vi "Get Typedef Path Dialog.vi"() -> (2 "Continue":bool, 3 "Stub VI Path":path, 5 "Typedef Path":path)   [LabVIEW 2012, in "Build Cluster of References__RCF.lvlib"]
uses:
  Build Cluster of References__RCF.lvlib
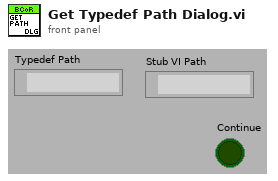
[diagram p1: front panel]
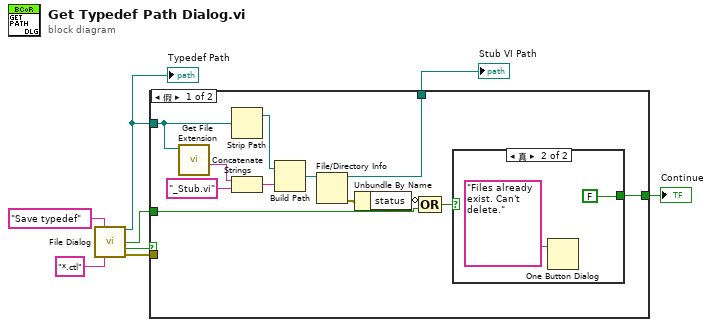
[diagram p0: block diagram]
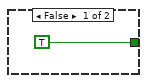
[diagram p2: hidden frame]
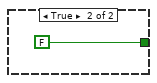
[diagram p3: hidden frame]
diagram:
  n1 = call "File Dialog"("prompt"="Save typedef", "pattern (all files)"="*.ctl") -> ("selected path"=w3:path, "exists"=w4:bool, "cancelled"=w6:bool, "error out"=w5:errorcluster)  [unwired: 5 in, 5 out]
  "Typedef Path" <- w3
  n2 = case shown="假" w6 {
    tunnel: w5 -> [_ _]
    tunnel: w4 -> [w20 _]
    tunnel: w3 -> [w16 _]
    tunnel: [w10 FALSE] -> w2
    tunnel: [w9 _] -> w1
    frame False {
      n3 = call <vilib>:"Get File Extension.vi"("file"=w16) -> ("filename without extension"=w19:string)  [unwired: 1 in, 9 out]
      n4 = Strip Path(path=w16) -> (stripped path=w17:path)  [unwired: 1 out]
      n5 = Concatenate Strings(w19, "_Stub.vi" ("string")) -> (w15:string)
      n6 = Build Path(base path=w17, name or relative path=w15) -> (appended path=w14:path)
      n7 = File/Directory Info(path=w14) -> (path out=w9:path, error out=w13:errorcluster)  [unwired: 1 in, 5 out]
      n8 = Unbundle By Name(w13) -> ("status"=w12:bool)
      n9 = Compound Arithmetic op=OR(invert w12, w20) -> (w11:bool)
      n10 = case shown="真" w11 {
        tunnel: [TRUE ("T button?") FALSE ("T button?")] -> w10
        frame False {
        }
        frame True {
          n11 = One Button Dialog(message="Files already exist. Can't delete.") -> ()  [unwired: 2 out]
        }
      }
    }
    frame True {
    }
  }
  "Continue" <- w2
  "Stub VI Path" <- w1
